vi "Vertical Insert 3.vi"(4 "Side":T1=enum."right", 7 "MaxAngle":dbl=40.0, 8 "error in":errorcluster, 9 "Speed":dbl=10.0, 10 "depth":dbl, 11 "deg/mm":dbl=10.0) -> (0 "error out":errorcluster)   [LabVIEW 2013]
uses:
  ROS/Code/SubVIs/BaxterSide.ctl
  ROS/Code/Console/Servers/ServerSubs/(nist) Arm Globals.vi
  Prim/Fwd Kenimatics - array.vi
  <vilib>/Analysis/Matrix/Numeric/Multiply/Multiply - RM,RM.vi
  Move Matrix.vi
  <vilib>/Analysis/Matrix/NI_Matrix.lvlib
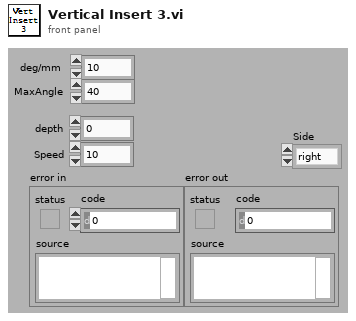
[diagram p1: front panel]
types:
  T1 = typedef "BaxterSide.ctl" = enum16{"left", "right"}
  T2 = typedef "NI_Matrix.lvlib/RealMatrix.ctl" = dbl[][]
  T3 = cluster{"X":dbl, "Y":dbl, "Z":dbl, "Roll":dbl, "Pitch":dbl, "Yaw":dbl}
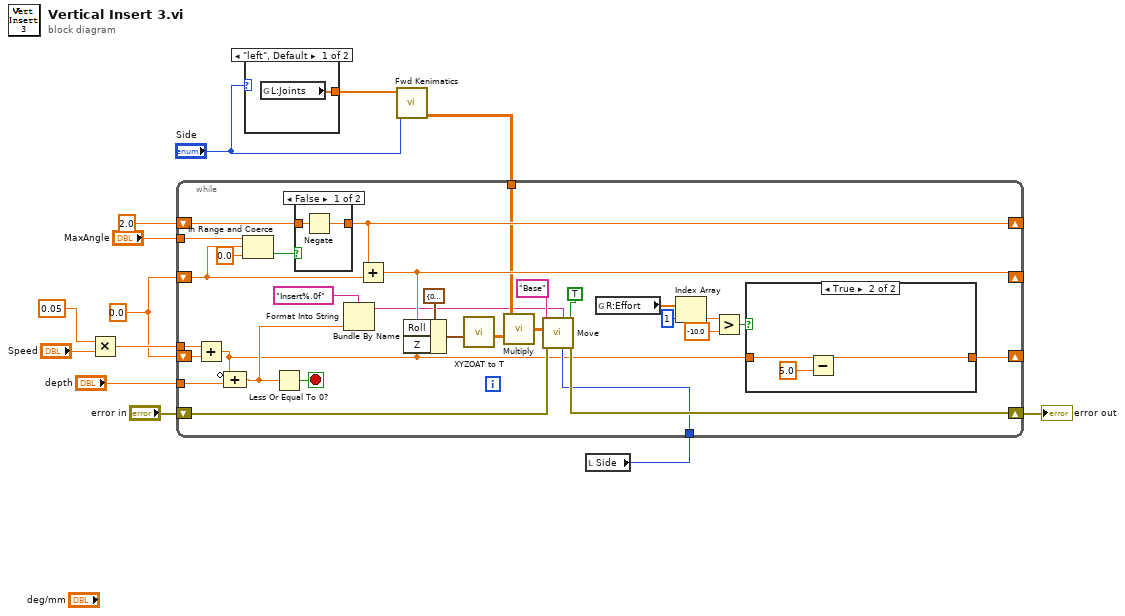
[diagram p0: block diagram]
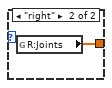
[diagram p4: hidden frame]
diagram:
  w5 = 0.0
  n1 = Multiply(x=0.05 ("y"), y="Speed") -> (x*y=w8:dbl)
  n2 = case shown="\"left\", Default" "Side" {
    tunnel: [w14 w15] -> w13
    frame "left", Default {
      n3 = global read "(nist) Arm Globals.vi" "L:Joints"() -> (w14:dbl[])
    }
    frame "right" {
      n4 = global read "(nist) Arm Globals.vi" "R:Joints"() -> (w15:dbl[])
    }
  }
  n5 = call-poly "Fwd Kenimatics.vi"("Side"="Side", "Joints"=w13) -> ("Matrix"=w6:T2)  [unwired: 8 in, 1 out]
  n6 = local read "Side"() -> (w1:T1)
  n7 = while {
    tunnel: "depth" -> [w46]
    shift-right: [w16] -> _
    shift-left: w5 -> [w45]
    tunnel: w8 -> [w44]
    shift-right: [w38] -> _
    shift-left: 2.0 -> [w42]
    tunnel: "MaxAngle" -> [w40]
    shift-right: [w31] -> _
    shift-left: w5 -> [w39]
    tunnel: w6 -> [w30]
    shift-right: [w24] -> w2
    shift-left: "error in" -> [w25]
    tunnel: w1 -> [w23]
    stop <- w29 stop-if-true
    n8 = Add(x=w44, y=w45) -> (x+y=w17:dbl)
    n9 = Compound Arithmetic op=ADD(invert w17, w46) -> (w27:dbl)
    n10 = In Range and Coerce(upper limit=w40, x=w39, lower limit=0.0) -> (In Range?=w43:bool)  [unwired: 1 out]
    n11 = Less Or Equal To 0?(x=w27) -> (x <= 0?=w29:bool)
    n12 = case shown="False" w43 {
      tunnel: w42 -> [w52 w53]
      tunnel: [w51 w53] -> w38
      frame False {
        n13 = Negate(x=w52) -> (-x=w51:dbl)
      }
      frame True {
      }
    }
    n14 = Format Into String(format string="Insert%.0f", w27) -> (resulting string=w26:string)  [unwired: 2 in, 1 out]
    n15 = Add(x=w38, y=w39) -> (x+y=w31:dbl)
    n16 = Bundle By Name(cluster=T3 {"X"=0.0, "Y"=0.0, "Z"=0.0, "Roll"=0.0, "Pitch"=0.0, "Yaw"=0.0} ("XYZOAT"), "Roll"=w31, "Z"=w17) -> (w32:T3)
    n17 = call "XYZOAT to T.vi"("XYZOAT"=w32) -> ("T"=w33:T2)  [unwired: 10 in]
    n18 = call-poly <vilib>:"Multiply.vi"("Real Matrix B"=w33, "Real Matrix A"=w30) -> ("A * B"=w35:T2)
    n19 = call-poly "Move.vi"("Make Vertical"=TRUE, "Side"=w23, "Label"=w26, "error in"=w25, "Offset"=w35, "Location"="Base") -> ("error out"=w24:errorcluster)  [unwired: 5 in]
    n20 = global read "(nist) Arm Globals.vi" "R:Effort"() -> (w22:dbl[])
    n21 = Index Array(array=w22, index=1) -> (element=w20:dbl)
    n22 = Greater?(x=w20, y=-10.0) -> (0:w18:bool)
    n23 = case shown="True" w18 {
      tunnel: w17 -> [w47 w50]
      tunnel: [w47 w49] -> w16
      frame False {
      }
      frame True {
        n24 = Subtract(x=w50, y=5.0) -> (x-y=w49:dbl)
      }
    }
  }
  "error out" <- w2
